vi "Schedule.vi"(8 "error in (no error)":errorcluster, 10 "scheduling":i32, 11 "MQTT-Client in":refnum<class "MQTT-Client.lvclass">) -> (0 "error out":errorcluster, 3 "MQTT-Client out":refnum<class "MQTT-Client.lvclass">)   [LabVIEW 2023, in "MQTT-Client.lvlib" / "MQTT-Client.lvclass"]
uses:
  MQTT-Client.lvclass
  MQTT-Client.lvclass/MQTT-Client.ctl
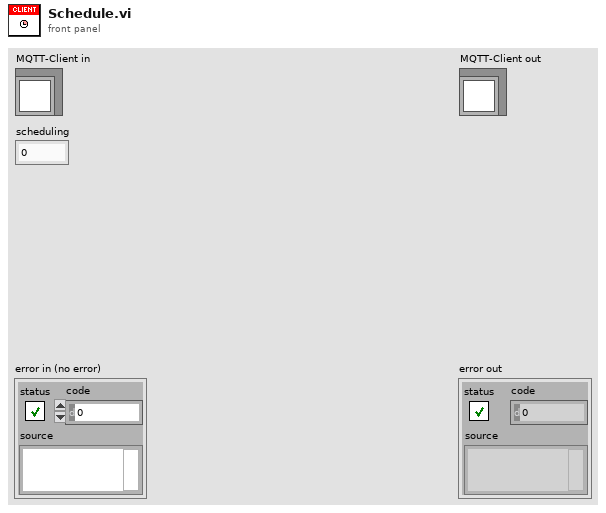
[diagram p1: front panel]
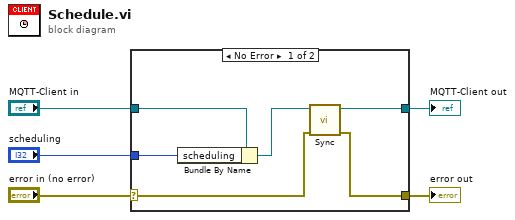
[diagram p0: block diagram]
diagram:
  n1 = case shown="No Error" "error in (no error)" {
    selector: "error in (no error)" -> [w7 w13]
    tunnel: [w6 w13] -> w4
    tunnel: [w11 w12] -> w2
    tunnel: "MQTT-Client in" -> [w9 w12]
    tunnel: "scheduling" -> [w10 _]
    frame No Error {
      n2 = Bundle By Name(cluster=w9, "scheduling"=w10) -> (w8:refnum<class "MQTT-Client.lvclass">)
      n3 = call "Sync.vi"("error in (no error)"=w7, "MQTT-Client in"=w8) -> ("error out"=w6:errorcluster, "MQTT-Client out"=w11:refnum<class "MQTT-Client.lvclass">)  [unwired: 8 in]
    }
    frame Error {
    }
  }
  "error out" <- w4
  "MQTT-Client out" <- w2
